vi "Run.vi"(7 "Team Index":i32, 8 "Column":i32, 9 "Row":i32, 10 "View":i32[](array[numeric]) caption="View (Team Index, -1: empty)", 11 "Expand in":refnum<class "Cautious Wolf.lvclass">) -> (0 "Replicated":refnum<class "Square.lvclass">, 1 "Direction":T1, 2 "Action":T2, 3 "Square Out":refnum<class "Square.lvclass">)   [LabVIEW 2015, in "Cautious Wolf.lvclass"]
uses:
  Cautious Wolf.lvclass
  Square/Square.lvclass
  Type Defs/Action Enum.ctl
  Type Defs/Direction Enum.ctl
  Cautious Wolf.lvclass/Cautious Wolf.ctl
  SubVIs/Read-Only Globals.vi
  SubVIs/Globals (private).vi
  Type Defs/SB Type Defs.lvlib
panel:
  # "NW\nN\nNE\nE\nSE\nS\nSW\nW"
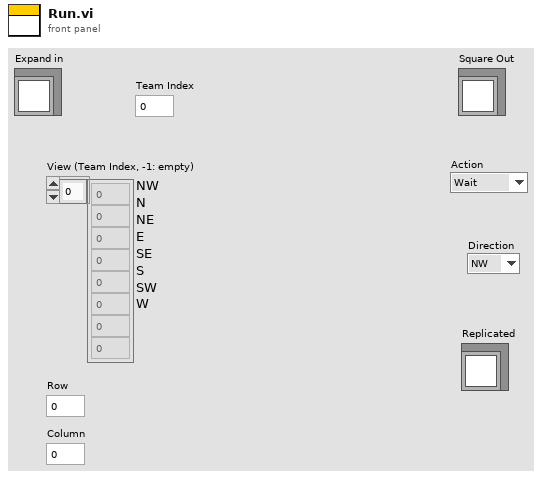
[diagram p1: front panel]
types:
  T1 = typedef "SB Type Defs.lvlib/Direction Enum.ctl" = enum16{"NW", "N", "NE", "E", "SE", "S", "SW", "W"}
  T2 = typedef "SB Type Defs.lvlib/Action Enum.ctl" = enum16{"Wait", "Move", "Attack", "Replicate"}
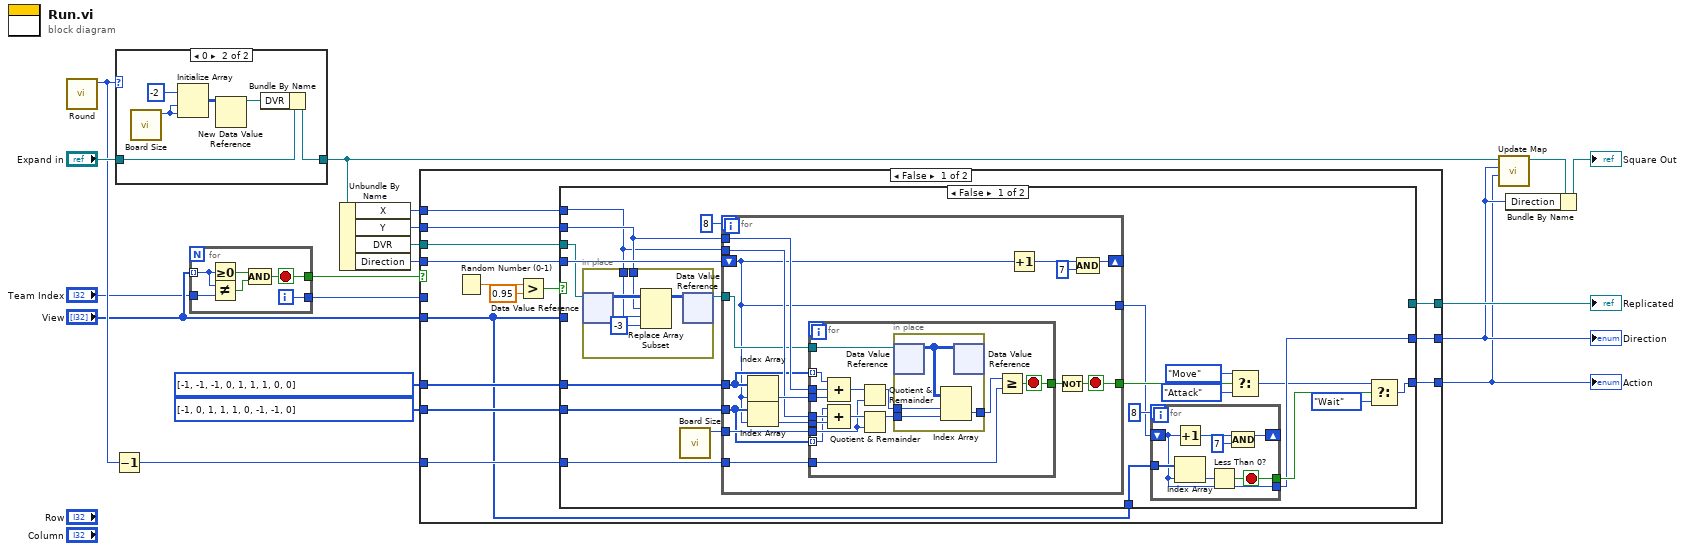
[diagram p0: block diagram]
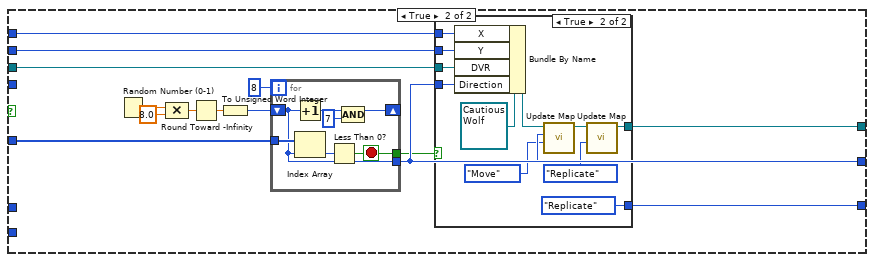
[diagram p3: hidden frame]
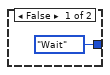
[diagram p4: hidden frame]
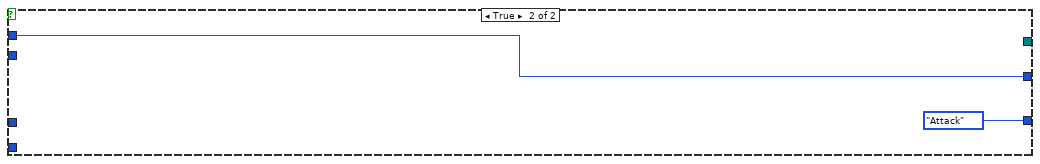
[diagram p5: hidden frame]
diagram:
  n1 = call "Round.vi"() -> ("Round"=w6:i32)  [unwired: 11 in]
  n2 = Decrement(x=w6) -> (x-1=w5:i32)
  n3 = case shown="0" w6 {
    tunnel: "Expand in" -> [w20 w24]
    tunnel: [w20 w22] -> w13
    frame Default {
    }
    frame 0 {
      n4 = call "Board Size.vi"() -> ("Board Size"=w21:i32)  [unwired: 11 in]
      n5 = Initialize Array(-2, w21, w21) -> (w25:i32[][])
      n6 = New Data Value Reference(data value=w25) -> (data value reference=w23:refnum<data-value>)  [unwired: 1 in, 1 out]
      n7 = Bundle By Name(cluster=w24, "DVR"=w23) -> (w22:refnum<class "Cautious Wolf.lvclass">)
    }
  }
  n8 = for {
    tunnel: "View" -> [w30] mode=indexing
    tunnel: "Team Index" -> [w31]
    tunnel: [w28] -> w1
    tunnel: [w27] -> w2
    i -> [w28]
    stop <- w27 stop-if-true
    n9 = Greater Or Equal To 0?(x=w30) -> (x >= 0?=w32:bool)
    n10 = Not Equal?(x=w30, y=w31) -> (x != y?=w29:bool)
    n11 = Compound Arithmetic op=AND(w32, w29) -> (w27:bool)
  }
  n12 = Unbundle By Name(w13) -> ("X"=w9:i32, "Y"=w10:i32, "DVR"=w15:refnum<data-value>, "Direction"=w17:T1)
  n13 = case shown="False" w2 {
    tunnel: [w42 w147] -> w12
    tunnel: [w46 Action_Enum."Attack" ("Action")] -> w11
    tunnel: "View" -> [w33 _]
    tunnel: [w45 _] -> w19
    tunnel: w17 -> [w37 _]
    tunnel: w15 -> [w40 _]
    tunnel: w10 -> [w39 _]
    tunnel: w9 -> [w38 _]
    tunnel: i32[] [-1, -1, -1, 0, 1, 1, 1, 0, 0] -> [w36 _]
    tunnel: i32[] [-1, 0, 1, 1, 1, 0, -1, -1, 0] -> [w35 _]
    tunnel: w5 -> [w34 _]
    tunnel: w1 -> [_ w147]
    frame False {
      n14 = Random Number (0-1)() -> (number: 0 to 1=w43:dbl)
      n15 = Greater?(x=w43, y=0.95) -> (0:w41:bool)
      n16 = case shown="False" w41 {
        tunnel: [w47 w127] -> w46
        tunnel: [_ w115] -> w45
        tunnel: w33 -> [_ w125]
        tunnel: [w50 w116] -> w42
        tunnel: w40 -> [w62 w119]
        tunnel: w39 -> [w61 w118]
        tunnel: w38 -> [w60 w117]
        tunnel: w37 -> [w66 _]
        tunnel: w36 -> [w64 _]
        tunnel: w35 -> [w65 _]
        tunnel: w34 -> [w58 _]
        tunnel: w33 -> [w54 _]
        frame False {
          n17 = in-place {
            in-place-border: w61 -> [w77]
            in-place-border: w60 -> [w76]
            n18 = in-place-dvr #1(w62) -> (w79:i32[][])  [unwired: 1 out]
            n19 = Replace Array Subset(array=w79, new element=-3 ("new element/subarray"), index (row)=w77, index (col)=w76) -> (w78:i32[][])
            n20 = in-place-dvr #1(w78) -> (w59:refnum<data-value>)  [unwired: 1 out]
          }
          n21 = call "Board Size.vi"() -> ("Board Size"=w63:i32)  [unwired: 11 in]
          n22 = for {
            N: 8 -> [_]
            shift-right: [w92] -> _
            shift-left: w66 -> [w80]
            tunnel: w65 -> [w85]
            tunnel: w64 -> [w86]
            tunnel: w63 -> [w89]
            tunnel: w61 -> [w88]
            tunnel: w60 -> [w87]
            tunnel: w59 -> [w83]
            tunnel: w58 -> [w84]
            tunnel: [w81] -> w57
            tunnel: [w80] -> w53
            stop <- w81 stop-if-true
            n23 = Index Array(array=w86, index=w80) -> (element=w91:i32)
            n24 = Index Array(array=w85, index=w80) -> (element=w90:i32)
            n25 = for {
              tunnel: w91 -> [w107]
              tunnel: w90 -> [w106]
              tunnel: w89 -> [w105]
              tunnel: w88 -> [w104]
              tunnel: w87 -> [w103]
              tunnel: w86 -> [w102] mode=indexing
              tunnel: w85 -> [w101] mode=indexing
              tunnel: w84 -> [w96]
              tunnel: w83 -> [w100]
              tunnel: [w95] -> w82
              stop <- w95 stop-if-true
              n26 = Compound Arithmetic op=ADD(w102, w104, w107) -> (w108:i32)
              n27 = Compound Arithmetic op=ADD(w101, w103, w106) -> (w109:i32)
              n28 = Quotient & Remainder(x=w108, y=w105) -> (x-y*floor(x/y)=w99:i32)  [unwired: 1 out]
              n29 = Quotient & Remainder(x=w109, y=w105) -> (x-y*floor(x/y)=w98:i32)  [unwired: 1 out]
              n30 = in-place {
                in-place-border: w99 -> [w112]
                in-place-border: w98 -> [w111]
                in-place-border: [w110] -> w97
                n31 = in-place-dvr #2(w100) -> (w113:i32[][])  [unwired: 1 out]
                n32 = Index Array(array=w113, index (row)=w112, index (col)=w111) -> (element=w110:i32)
                n33 = in-place-dvr #2(w113) -> ()  [unwired: 2 out]
              }
              n34 = Greater Or Equal?(x=w97, y=w96) -> (x >= y?=w95:bool)
            }
            n35 = Increment(x=w80) -> (x+1=w94:i32)
            n36 = Not(x=w82) -> (.not. x?=w81:bool)
            n37 = Compound Arithmetic op=AND(w94, 7) -> (w92:i32)
          }
          n38 = for {
            N: 8 -> [_]
            tunnel: w54 -> [w74]
            shift-right: [w68] -> _
            shift-left: w53 -> [w72]
            tunnel: [w72] -> w50
            tunnel: [w71] -> w52
            stop <- w71 stop-if-true
            n39 = Increment(x=w72) -> (x+1=w69:i32)
            n40 = Index Array(array=w74, index=w72) -> (element=w73:i32)
            n41 = Less Than 0?(x=w73) -> (x < 0?=w71:bool)
            n42 = Compound Arithmetic op=AND(w69, 7) -> (w68:i32)
          }
          n43 = Select(t=Action_Enum."Move" ("y"), s=w57, f=Action_Enum."Attack" ("y")) -> (s? t:f=w48:T2)
          n44 = Select(t=w48, s=w52, f=Action_Enum."Wait" ("y")) -> (s? t:f=w47:T2)
        }
        frame True {
          n45 = Random Number (0-1)() -> (number: 0 to 1=w121:dbl)
          n46 = Compound Arithmetic op=MULTIPLY(w121, 8.0 ("value")) -> (w123:dbl)
          n47 = Round Toward -Infinity(1:w123) -> (0:w124:dbl)
          n48 = To Unsigned Word Integer(number=w124) -> (unsigned 16bit integer=w120:u16)
          n49 = for {
            N: 8 -> [_]
            tunnel: w125 -> [w146]
            shift-right: [w140] -> _
            shift-left: w120 -> [w144]
            tunnel: [w144] -> w116
            tunnel: [w143] -> w114
            stop <- w143 stop-if-true
            n50 = Increment(x=w144) -> (x+1=w141:u16)
            n51 = Index Array(array=w146, index=w144) -> (element=w145:i32)
            n52 = Less Than 0?(x=w145) -> (x < 0?=w143:bool)
            n53 = Compound Arithmetic op=AND(w141, u16 7 ("x+1")) -> (w140:u16)
          }
          n54 = case shown="True" w114 {
            tunnel: [Action_Enum."Wait" ("y") Action_Enum."Replicate" ("y")] -> w127
            tunnel: w119 -> [_ w137]
            tunnel: w118 -> [_ w136]
            tunnel: w117 -> [_ w135]
            tunnel: w116 -> [_ w133]
            tunnel: [_ w130] -> w115
            frame False {
            }
            frame True {
              n55 = Bundle By Name(cluster=refnum<class "Cautious Wolf.lvclass"> refnum ("Lone Wolf.lvclass"), "X"=w135, "Y"=w136, "DVR"=w137, "Direction"=w133) -> (w134:refnum<class "Cautious Wolf.lvclass">)
              n56 = call "Update Map.vi"("Action"=Action_Enum."Move", "Direction"=w133, "Class"=w134) -> ("Class"=w131:refnum<class "Cautious Wolf.lvclass">)  [unwired: 8 in]
              n57 = call "Update Map.vi"("Action"=Action_Enum."Replicate", "Class"=w131) -> ("Class"=w130:refnum<class "Cautious Wolf.lvclass">)  [unwired: 9 in]
            }
          }
        }
      }
    }
    frame True {
    }
  }
  "Action" <- w11
  "Direction" <- w12
  "Replicated" <- w19
  n58 = call "Update Map.vi"("Action"=w11, "Direction"=w12, "Class"=w13) -> ("Class"=w14:refnum<class "Cautious Wolf.lvclass">)  [unwired: 8 in]
  n59 = Bundle By Name(cluster=w14, "Direction"=w12) -> (→"Square Out":refnum<class "Cautious Wolf.lvclass">)
